vi "查询上序合格.vi"(8 "error in (no error)":errorcluster, 11 "产品ID":string="123456") -> (0 "error out":errorcluster, 1 "本序已做":bool, 2 "上序合格":bool)   [LabVIEW 2013]
uses:
  <vilib>/Utility/error.llb/whitespace.ctl
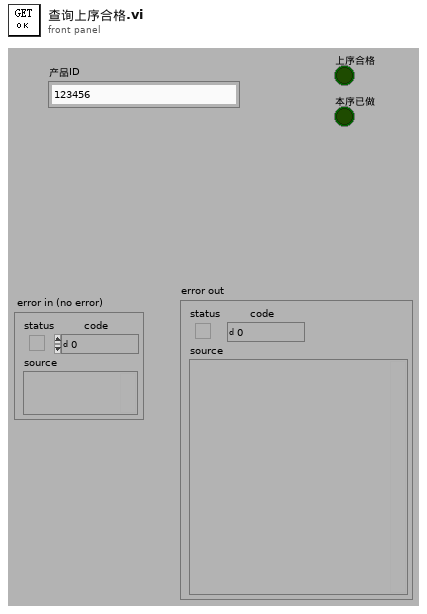
[diagram p1: front panel]
types:
  T1 = typedef "whitespace.ctl" = u16
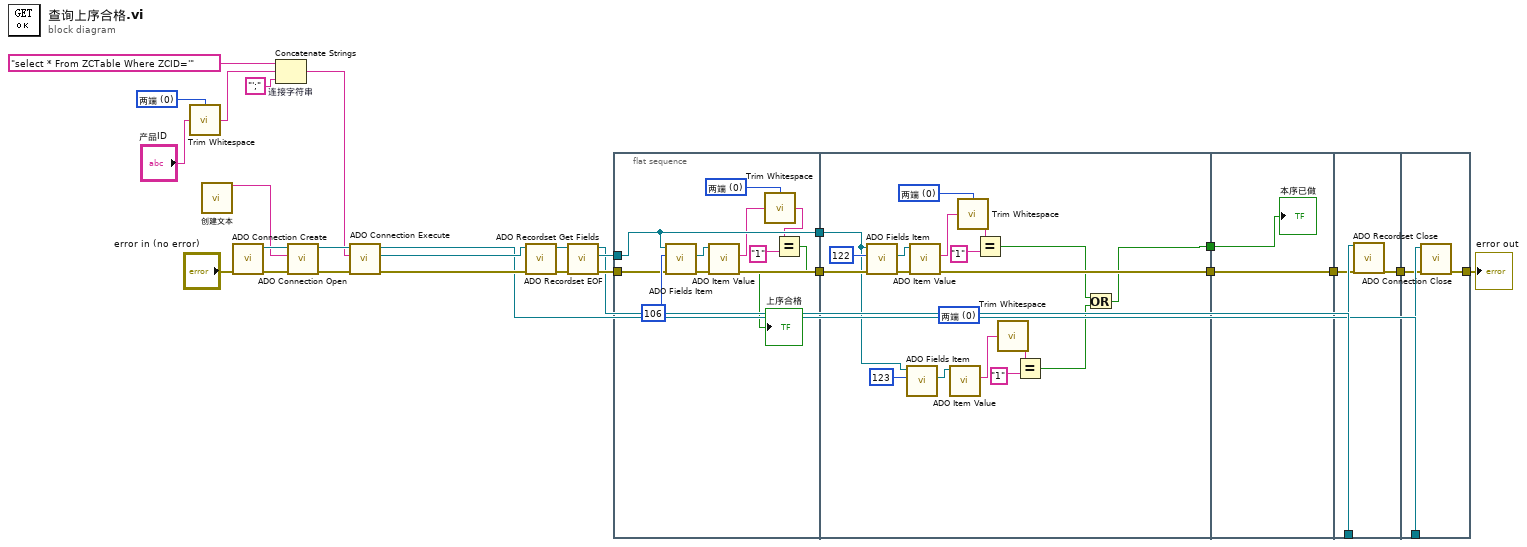
[diagram p0: block diagram]
diagram:
  w17 = T1 0 items=["两端", "字符串首端", "字符串末端"] ("location (both)")
  n1 = call <vilib>:"Trim Whitespace.vi"("string"="产品ID", "location (both)"=w17) -> ("trimmed string"=w18:string)
  n2 = call "创建文本"() -> ("Result"=w3:string)  [unwired: 14 in, 1 out]
  n3 = call "ADO Connection Create.vi"("error in (no error)"="error in (no error)") -> ("error out"=w26:errorcluster, "ADODB._Connection Out"=w27:refnum<k7>)  [unwired: 9 out]
  n4 = Concatenate Strings "连接字符串"("select * From ZCTable Where ZCID='" ("字符串 2"), w18, "';" ("字符串 2")) -> (w16:string)
  n5 = call "ADO Connection Open.vi"("error in (no error)"=w26, "ConnectionString"=w3, "ADODB._Connection In"=w27) -> ("error out"=w25:errorcluster, "ADODB._Connection Out"=w24:refnum<k7>)  [unwired: 7 out]
  n6 = call "ADO Connection Execute.vi"("error in (no error)"=w25, "CommandText"=w16, "ADODB._Connection In"=w24) -> ("error out"=w22:errorcluster, "RecordSet"=w23:refnum<k7>, "ADODB._Connection Out"=w8:refnum<k7>)  [unwired: 6 out]
  n7 = call "ADO Recordset EOF.vi"("error in (no error)"=w22, "ADODB._Recordset In"=w23) -> ("error out"=w13:errorcluster, "ADODB._Recordset Out"=w14:refnum<k7>)  [unwired: 8 out]
  n8 = call "ADO Recordset Get Fields.vi"("error in (no error)"=w13, "ADODB._Recordset In"=w14) -> ("error out"=w11:errorcluster, "Fields Out"=w12:refnum<k7>, "ADODB._Recordset Out"=w9:refnum<k7>)  [unwired: 7 out]
  n9 = flat-sequence {
    tunnel: w12 -> [w33]
    tunnel: w11 -> [w34]
    tunnel: [w38] -> w5
    tunnel: [w33] -> w4
    tunnel: w4 -> [w42]
    tunnel: w5 -> [w53]
    tunnel: [w48] -> w2
    tunnel: [w39] -> w1
    tunnel: [w58] -> w10
    tunnel: w2 -> [w58]
    tunnel: w1 -> [w57]
    tunnel: w10 -> [w60]
    tunnel: w9 -> [w61]
    tunnel: [w59] -> w7
    tunnel: w8 -> [w64]
    tunnel: w7 -> [w63]
    tunnel: [w62] -> w6
    frame #0 {
      w31 = T1 0 items=["两端", "字符串首端", "字符串末端"] ("location (both)")
      n10 = call "ADO Fields Item.vi"("error in (no error)"=w34, "Index"=106, "Fields In"=w33) -> ("error out"=w36:errorcluster, "Item Out"=w35:refnum<k7>)  [unwired: 7 out]
      n11 = call "ADO Item Value.vi"("error in (no error)"=w36, "Item In"=w35) -> ("error out"=w38:errorcluster, "Value"=w30:string)  [unwired: 8 out]
      n12 = call <vilib>:"Trim Whitespace.vi"("string"=w30, "location (both)"=w31) -> ("trimmed string"=w29:string)
      n13 = Equal?(x=w29, y="1") -> (x = y?=→"上序合格":bool)
    }
    frame #1 {
      (unwired) T1 0 items=["两端", "字符串首端", "字符串末端"] ("location (both)")
      w51 = T1 0 items=["两端", "字符串首端", "字符串末端"] ("location (both)")
      n14 = call "ADO Fields Item.vi"("error in (no error)"=w53, "Index"=122, "Fields In"=w42) -> ("error out"=w55:errorcluster, "Item Out"=w54:refnum<k7>)  [unwired: 7 out]
      n15 = call "ADO Fields Item.vi"("Index"=123, "Fields In"=w42) -> ("Item Out"=w44:refnum<k7>)  [unwired: 1 in, 8 out]
      n16 = call "ADO Item Value.vi"("error in (no error)"=w55, "Item In"=w54) -> ("error out"=w48:errorcluster, "Value"=w50:string)  [unwired: 8 out]
      n17 = call "ADO Item Value.vi"("Item In"=w44) -> ("Value"=w46:string)  [unwired: 1 in, 9 out]
      n18 = call <vilib>:"Trim Whitespace.vi"("string"=w50, "location (both)"=w51) -> ("trimmed string"=w49:string)
      n19 = Equal?(x=w49, y="1") -> (x = y?=w41:bool)
      n20 = call <vilib>:"Trim Whitespace.vi"("string"=w46) -> ("trimmed string"=w47:string)  [unwired: 1 in]
      n21 = Equal?(x=w47, y="1") -> (x = y?=w40:bool)
      n22 = Or(x=w41, y=w40) -> (x .or. y?=w39:bool)
    }
    frame #2 {
      "本序已做" <- w57
    }
    frame #3 {
      n23 = call "ADO Recordset Close.vi"("ADODB._Recordset In"=w61, "error in (no error)"=w60) -> ("error out"=w59:errorcluster)  [unwired: 17 out]
    }
    frame #4 {
      n24 = call "ADO Connection Close.vi"("error in (no error)"=w63, "ADODB._Connection In"=w64) -> ("error out"=w62:errorcluster)  [unwired: 9 out]
    }
  }
  "error out" <- w6
